vi "Self Event Alias.vi"(11 "TEMPLATE Event in":refnum<class "TEMPLATE Event.lvclass">) -> (2 "Self Event Alias":string)   [LabVIEW 2021, in "_Template.lvlib" / "Templates.lvlib" / "TEM Event.lvlib" / "TEMPLATE Event.lvclass"]
uses:
  TEMPLATE Event.lvclass
  TEMPLATE Event.lvclass/TEMPLATE Event.ctl
  <vilib>/Nathan Davis/jettl/jettl/Event/Event.lvclass
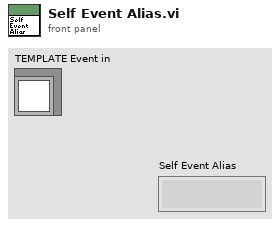
[diagram p1: front panel]
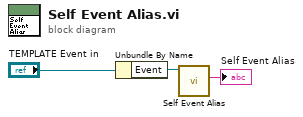
[diagram p0: block diagram]
diagram:
  n1 = Unbundle By Name("TEMPLATE Event in") -> ("Event"=w2:refnum<class "Event.lvclass">)
  n2 = call-dynamic "Self Event Alias.vi"("Event in"=w2) -> ("Self Event Alias"=→"Self Event Alias":string)  [unwired: 10 in]
